vi "getList.vi"(0 "SEDSpectrometer in":refnum<class "FiberSpectrograph.lvclass">, 5 "ListSizeInput":u32, 7 "RequiredSizeInput":u32, 9 "ListInpit":u8[](array[numeric]), 11 "error in (no error)":errorcluster) -> (4 "SEDSpectrometer out":refnum<class "FiberSpectrograph.lvclass">, 10 "List Output":u8[](array[numeric]), 15 "error out":errorcluster)   [LabVIEW 2016, in "FiberSpectrograph.lvclass"]
uses:
  FiberSpectrograph.lvclass
panel:
  out "RequiredSizeOutput":u32
  out "ListSizeOutput":u32
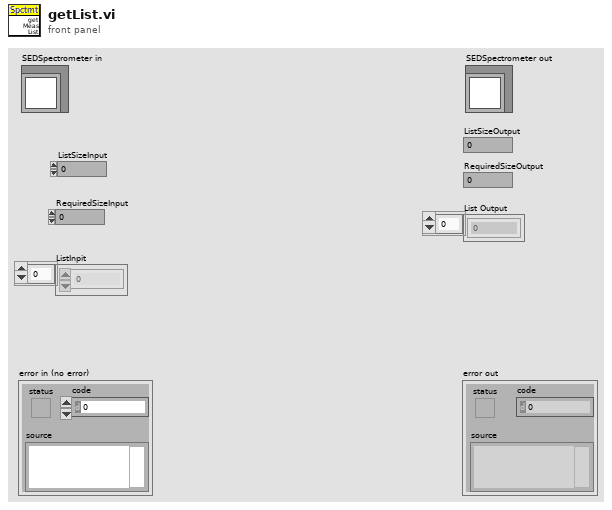
[diagram p1: front panel]
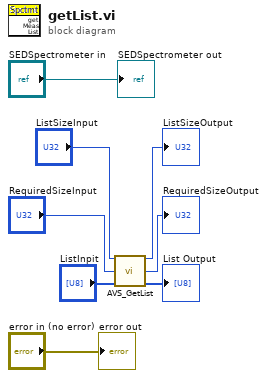
[diagram p0: block diagram]
diagram:
  n1 = call "AVS_GetList.vi"("ListSizeInput"="ListSizeInput", "RequiredSizeInput"="RequiredSizeInput", "ListInpit"="ListInpit") -> ("ListSizeOutput"=→"ListSizeOutput":u32, "RequiredSizeOutput"=→"RequiredSizeOutput":u32, "List Output"=→"List Output":u8[])  [unwired: 10 in]
  "error out" <- "error in (no error)"
  "SEDSpectrometer out" <- "SEDSpectrometer in"
